vi "Set Dev Notice Event.vi"(8 "error in (no error)":errorcluster, 10 "rmvevent":u32, 11 "addevent":u32) -> (0 "error out":errorcluster, 2 "rmvevent out":u32, 3 "addevent out":u32)   [LabVIEW 2021, in "vmmsolib.lvlib"]
doc: "DLL_API void WINAPI SetDevNoticeEvent(HANDLE addevent, HANDLE rmvevent);"
uses:
  vmmsolib.lvlib
  vmmso.dll
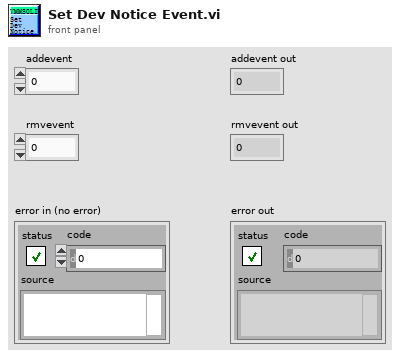
[diagram p1: front panel]
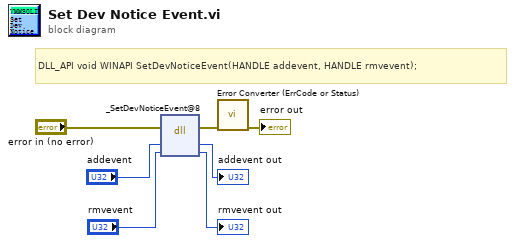
[diagram p0: block diagram]
diagram:
  # "DLL_API void WINAPI SetDevNoticeEvent(HANDLE addevent, HANDLE rmvevent);"
  n1 = dll-call lib="D:/VmMsoSDK/demo-Labview/2021/vmmsolib/vmmso.*" fn="_SetDevNoticeEvent@8"(error in="error in (no error)", "addevent"="addevent", "rmvevent"="rmvevent") -> (error out=w2:errorcluster, "addevent"=→"addevent out":u32, "rmvevent"=→"rmvevent out":u32)  [unwired: 3 in, 1 out]
  n2 = call "Error Converter (ErrCode or Status).vi"("error in (no error)"=w2) -> ("error out"=→"error out":errorcluster)  [unwired: 10 in]
